vi "Auto.vi"   [LabVIEW 2017]
uses:
  <userlib>/836-Library/System/QCP_V2/QCPSupportCode/QCPData.ctl
  <userlib>/836-Library/System/QCP_V2/QCPSupportCode/QCP_GetDblArr.vi
  <userlib>/836-Library/System/QCP_V2/QCPSupportCode/QCP_GetDbl.vi
types:
  T1 = typedef "Semaphore RefNum" = refnum<k1>
  T2 = cluster{"Data Value Refnum":refnum<data-value>, "semaphore":T1}
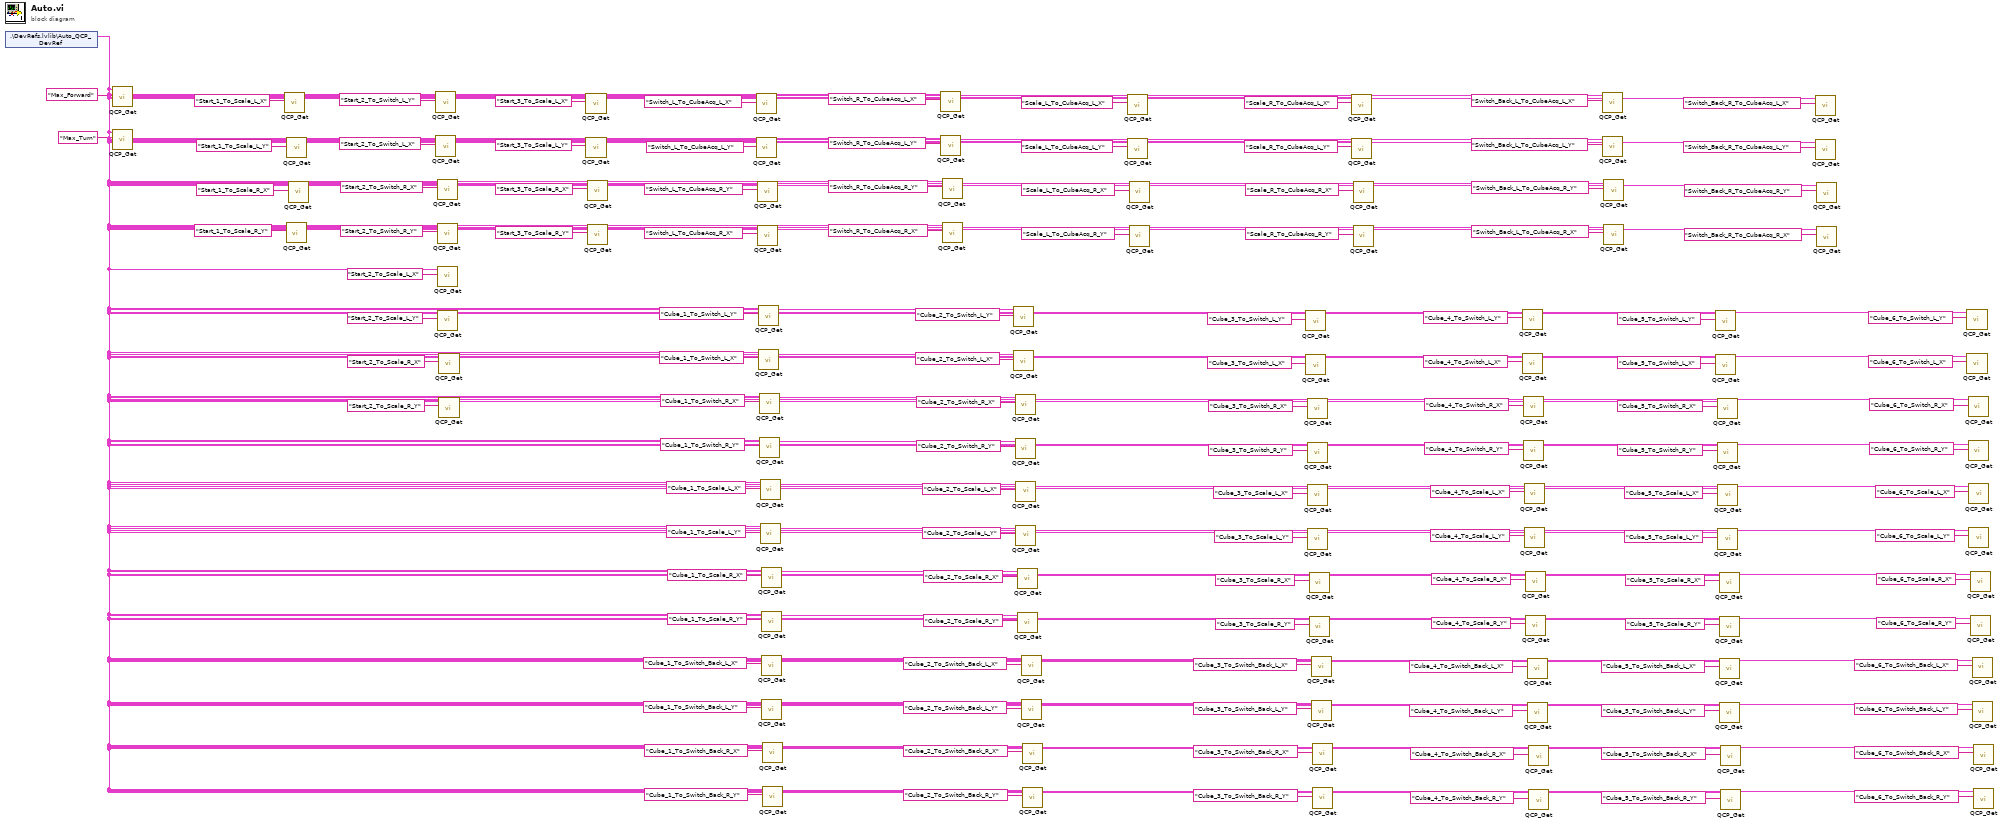
[diagram p0: block diagram]
diagram:
  n1 = shared-variable ".\\DevRefs.lvlib\\Auto_QCP_DevRef"() -> (w1:T2)  [unwired: 1 in, 1 out]
  n2 = call-poly <userlib>:"QCP_Get.vi"("Value Name"="Max_Forward", "QCP_DevRef_In"=w1) -> ()  [unwired: 7 in, 3 out]
  n3 = call-poly <userlib>:"QCP_Get.vi"("Value Name"="Max_Turn", "QCP_DevRef_In"=w1) -> ()  [unwired: 7 in, 3 out]
  n4 = call-poly <userlib>:"QCP_Get.vi"("Value Name"="Start_1_To_Scale_L_X", "QCP_DevRef_In"=w1) -> ()  [unwired: 7 in, 3 out]
  n5 = call-poly <userlib>:"QCP_Get.vi"("Value Name"="Start_1_To_Scale_R_Y", "QCP_DevRef_In"=w1) -> ()  [unwired: 7 in, 3 out]
  n6 = call-poly <userlib>:"QCP_Get.vi"("Value Name"="Start_1_To_Scale_L_Y", "QCP_DevRef_In"=w1) -> ()  [unwired: 7 in, 3 out]
  n7 = call-poly <userlib>:"QCP_Get.vi"("Value Name"="Start_1_To_Scale_R_X", "QCP_DevRef_In"=w1) -> ()  [unwired: 7 in, 3 out]
  n8 = call-poly <userlib>:"QCP_Get.vi"("Value Name"="Start_2_To_Switch_L_Y", "QCP_DevRef_In"=w1) -> ()  [unwired: 7 in, 3 out]
  n9 = call-poly <userlib>:"QCP_Get.vi"("Value Name"="Start_2_To_Switch_L_X", "QCP_DevRef_In"=w1) -> ()  [unwired: 7 in, 3 out]
  n10 = call-poly <userlib>:"QCP_Get.vi"("Value Name"="Start_2_To_Switch_R_X", "QCP_DevRef_In"=w1) -> ()  [unwired: 7 in, 3 out]
  n11 = call-poly <userlib>:"QCP_Get.vi"("Value Name"="Start_2_To_Switch_R_Y", "QCP_DevRef_In"=w1) -> ()  [unwired: 7 in, 3 out]
  n12 = call-poly <userlib>:"QCP_Get.vi"("Value Name"="Start_2_To_Scale_L_X", "QCP_DevRef_In"=w1) -> ()  [unwired: 7 in, 3 out]
  n13 = call-poly <userlib>:"QCP_Get.vi"("Value Name"="Start_2_To_Scale_L_Y", "QCP_DevRef_In"=w1) -> ()  [unwired: 7 in, 3 out]
  n14 = call-poly <userlib>:"QCP_Get.vi"("Value Name"="Start_2_To_Scale_R_X", "QCP_DevRef_In"=w1) -> ()  [unwired: 7 in, 3 out]
  n15 = call-poly <userlib>:"QCP_Get.vi"("Value Name"="Start_2_To_Scale_R_Y", "QCP_DevRef_In"=w1) -> ()  [unwired: 7 in, 3 out]
  n16 = call-poly <userlib>:"QCP_Get.vi"("Value Name"="Start_3_To_Scale_L_X", "QCP_DevRef_In"=w1) -> ()  [unwired: 7 in, 3 out]
  n17 = call-poly <userlib>:"QCP_Get.vi"("Value Name"="Start_3_To_Scale_L_Y", "QCP_DevRef_In"=w1) -> ()  [unwired: 7 in, 3 out]
  n18 = call-poly <userlib>:"QCP_Get.vi"("Value Name"="Start_3_To_Scale_R_X", "QCP_DevRef_In"=w1) -> ()  [unwired: 7 in, 3 out]
  n19 = call-poly <userlib>:"QCP_Get.vi"("Value Name"="Start_3_To_Scale_R_Y", "QCP_DevRef_In"=w1) -> ()  [unwired: 7 in, 3 out]
  n20 = call-poly <userlib>:"QCP_Get.vi"("Value Name"="Switch_L_To_CubeAcq_L_X", "QCP_DevRef_In"=w1) -> ()  [unwired: 7 in, 3 out]
  n21 = call-poly <userlib>:"QCP_Get.vi"("Value Name"="Switch_L_To_CubeAcq_L_Y", "QCP_DevRef_In"=w1) -> ()  [unwired: 7 in, 3 out]
  n22 = call-poly <userlib>:"QCP_Get.vi"("Value Name"="Switch_L_To_CubeAcq_R_Y", "QCP_DevRef_In"=w1) -> ()  [unwired: 7 in, 3 out]
  n23 = call-poly <userlib>:"QCP_Get.vi"("Value Name"="Switch_L_To_CubeAcq_R_X", "QCP_DevRef_In"=w1) -> ()  [unwired: 7 in, 3 out]
  n24 = call-poly <userlib>:"QCP_Get.vi"("Value Name"="Cube_1_To_Switch_L_Y", "QCP_DevRef_In"=w1) -> ()  [unwired: 7 in, 3 out]
  n25 = call-poly <userlib>:"QCP_Get.vi"("Value Name"="Cube_1_To_Switch_L_X", "QCP_DevRef_In"=w1) -> ()  [unwired: 7 in, 3 out]
  n26 = call-poly <userlib>:"QCP_Get.vi"("Value Name"="Cube_1_To_Switch_R_X", "QCP_DevRef_In"=w1) -> ()  [unwired: 7 in, 3 out]
  n27 = call-poly <userlib>:"QCP_Get.vi"("Value Name"="Cube_1_To_Switch_R_Y", "QCP_DevRef_In"=w1) -> ()  [unwired: 7 in, 3 out]
  n28 = call-poly <userlib>:"QCP_Get.vi"("Value Name"="Cube_1_To_Scale_L_X", "QCP_DevRef_In"=w1) -> ()  [unwired: 7 in, 3 out]
  n29 = call-poly <userlib>:"QCP_Get.vi"("Value Name"="Cube_1_To_Scale_L_Y", "QCP_DevRef_In"=w1) -> ()  [unwired: 7 in, 3 out]
  n30 = call-poly <userlib>:"QCP_Get.vi"("Value Name"="Cube_1_To_Scale_R_X", "QCP_DevRef_In"=w1) -> ()  [unwired: 7 in, 3 out]
  n31 = call-poly <userlib>:"QCP_Get.vi"("Value Name"="Cube_1_To_Scale_R_Y", "QCP_DevRef_In"=w1) -> ()  [unwired: 7 in, 3 out]
  n32 = call-poly <userlib>:"QCP_Get.vi"("Value Name"="Cube_1_To_Switch_Back_L_X", "QCP_DevRef_In"=w1) -> ()  [unwired: 7 in, 3 out]
  n33 = call-poly <userlib>:"QCP_Get.vi"("Value Name"="Cube_1_To_Switch_Back_L_Y", "QCP_DevRef_In"=w1) -> ()  [unwired: 7 in, 3 out]
  n34 = call-poly <userlib>:"QCP_Get.vi"("Value Name"="Cube_1_To_Switch_Back_R_X", "QCP_DevRef_In"=w1) -> ()  [unwired: 7 in, 3 out]
  n35 = call-poly <userlib>:"QCP_Get.vi"("Value Name"="Cube_1_To_Switch_Back_R_Y", "QCP_DevRef_In"=w1) -> ()  [unwired: 7 in, 3 out]
  n36 = call-poly <userlib>:"QCP_Get.vi"("Value Name"="Switch_R_To_CubeAcq_L_X", "QCP_DevRef_In"=w1) -> ()  [unwired: 7 in, 3 out]
  n37 = call-poly <userlib>:"QCP_Get.vi"("Value Name"="Switch_R_To_CubeAcq_L_Y", "QCP_DevRef_In"=w1) -> ()  [unwired: 7 in, 3 out]
  n38 = call-poly <userlib>:"QCP_Get.vi"("Value Name"="Switch_R_To_CubeAcq_R_Y", "QCP_DevRef_In"=w1) -> ()  [unwired: 7 in, 3 out]
  n39 = call-poly <userlib>:"QCP_Get.vi"("Value Name"="Switch_R_To_CubeAcq_R_X", "QCP_DevRef_In"=w1) -> ()  [unwired: 7 in, 3 out]
  n40 = call-poly <userlib>:"QCP_Get.vi"("Value Name"="Cube_2_To_Switch_L_Y", "QCP_DevRef_In"=w1) -> ()  [unwired: 7 in, 3 out]
  n41 = call-poly <userlib>:"QCP_Get.vi"("Value Name"="Cube_2_To_Switch_L_X", "QCP_DevRef_In"=w1) -> ()  [unwired: 7 in, 3 out]
  n42 = call-poly <userlib>:"QCP_Get.vi"("Value Name"="Cube_2_To_Switch_R_X", "QCP_DevRef_In"=w1) -> ()  [unwired: 7 in, 3 out]
  n43 = call-poly <userlib>:"QCP_Get.vi"("Value Name"="Cube_2_To_Switch_R_Y", "QCP_DevRef_In"=w1) -> ()  [unwired: 7 in, 3 out]
  n44 = call-poly <userlib>:"QCP_Get.vi"("Value Name"="Cube_2_To_Scale_L_X", "QCP_DevRef_In"=w1) -> ()  [unwired: 7 in, 3 out]
  n45 = call-poly <userlib>:"QCP_Get.vi"("Value Name"="Cube_2_To_Scale_L_Y", "QCP_DevRef_In"=w1) -> ()  [unwired: 7 in, 3 out]
  n46 = call-poly <userlib>:"QCP_Get.vi"("Value Name"="Cube_2_To_Scale_R_X", "QCP_DevRef_In"=w1) -> ()  [unwired: 7 in, 3 out]
  n47 = call-poly <userlib>:"QCP_Get.vi"("Value Name"="Cube_2_To_Scale_R_Y", "QCP_DevRef_In"=w1) -> ()  [unwired: 7 in, 3 out]
  n48 = call-poly <userlib>:"QCP_Get.vi"("Value Name"="Cube_2_To_Switch_Back_L_X", "QCP_DevRef_In"=w1) -> ()  [unwired: 7 in, 3 out]
  n49 = call-poly <userlib>:"QCP_Get.vi"("Value Name"="Cube_2_To_Switch_Back_L_Y", "QCP_DevRef_In"=w1) -> ()  [unwired: 7 in, 3 out]
  n50 = call-poly <userlib>:"QCP_Get.vi"("Value Name"="Cube_2_To_Switch_Back_R_X", "QCP_DevRef_In"=w1) -> ()  [unwired: 7 in, 3 out]
  n51 = call-poly <userlib>:"QCP_Get.vi"("Value Name"="Cube_2_To_Switch_Back_R_Y", "QCP_DevRef_In"=w1) -> ()  [unwired: 7 in, 3 out]
  n52 = call-poly <userlib>:"QCP_Get.vi"("Value Name"="Scale_L_To_CubeAcq_L_X", "QCP_DevRef_In"=w1) -> ()  [unwired: 7 in, 3 out]
  n53 = call-poly <userlib>:"QCP_Get.vi"("Value Name"="Scale_L_To_CubeAcq_L_Y", "QCP_DevRef_In"=w1) -> ()  [unwired: 7 in, 3 out]
  n54 = call-poly <userlib>:"QCP_Get.vi"("Value Name"="Scale_L_To_CubeAcq_R_X", "QCP_DevRef_In"=w1) -> ()  [unwired: 7 in, 3 out]
  n55 = call-poly <userlib>:"QCP_Get.vi"("Value Name"="Scale_L_To_CubeAcq_R_Y", "QCP_DevRef_In"=w1) -> ()  [unwired: 7 in, 3 out]
  n56 = call-poly <userlib>:"QCP_Get.vi"("Value Name"="Cube_3_To_Switch_L_Y", "QCP_DevRef_In"=w1) -> ()  [unwired: 7 in, 3 out]
  n57 = call-poly <userlib>:"QCP_Get.vi"("Value Name"="Cube_3_To_Switch_L_X", "QCP_DevRef_In"=w1) -> ()  [unwired: 7 in, 3 out]
  n58 = call-poly <userlib>:"QCP_Get.vi"("Value Name"="Cube_3_To_Switch_R_X", "QCP_DevRef_In"=w1) -> ()  [unwired: 7 in, 3 out]
  n59 = call-poly <userlib>:"QCP_Get.vi"("Value Name"="Cube_3_To_Switch_R_Y", "QCP_DevRef_In"=w1) -> ()  [unwired: 7 in, 3 out]
  n60 = call-poly <userlib>:"QCP_Get.vi"("Value Name"="Cube_3_To_Scale_L_X", "QCP_DevRef_In"=w1) -> ()  [unwired: 7 in, 3 out]
  n61 = call-poly <userlib>:"QCP_Get.vi"("Value Name"="Cube_3_To_Scale_L_Y", "QCP_DevRef_In"=w1) -> ()  [unwired: 7 in, 3 out]
  n62 = call-poly <userlib>:"QCP_Get.vi"("Value Name"="Cube_3_To_Scale_R_X", "QCP_DevRef_In"=w1) -> ()  [unwired: 7 in, 3 out]
  n63 = call-poly <userlib>:"QCP_Get.vi"("Value Name"="Cube_3_To_Scale_R_Y", "QCP_DevRef_In"=w1) -> ()  [unwired: 7 in, 3 out]
  n64 = call-poly <userlib>:"QCP_Get.vi"("Value Name"="Cube_3_To_Switch_Back_L_X", "QCP_DevRef_In"=w1) -> ()  [unwired: 7 in, 3 out]
  n65 = call-poly <userlib>:"QCP_Get.vi"("Value Name"="Cube_3_To_Switch_Back_L_Y", "QCP_DevRef_In"=w1) -> ()  [unwired: 7 in, 3 out]
  n66 = call-poly <userlib>:"QCP_Get.vi"("Value Name"="Cube_3_To_Switch_Back_R_X", "QCP_DevRef_In"=w1) -> ()  [unwired: 7 in, 3 out]
  n67 = call-poly <userlib>:"QCP_Get.vi"("Value Name"="Cube_3_To_Switch_Back_R_Y", "QCP_DevRef_In"=w1) -> ()  [unwired: 7 in, 3 out]
  n68 = call-poly <userlib>:"QCP_Get.vi"("Value Name"="Scale_R_To_CubeAcq_L_X", "QCP_DevRef_In"=w1) -> ()  [unwired: 7 in, 3 out]
  n69 = call-poly <userlib>:"QCP_Get.vi"("Value Name"="Scale_R_To_CubeAcq_L_Y", "QCP_DevRef_In"=w1) -> ()  [unwired: 7 in, 3 out]
  n70 = call-poly <userlib>:"QCP_Get.vi"("Value Name"="Scale_R_To_CubeAcq_R_X", "QCP_DevRef_In"=w1) -> ()  [unwired: 7 in, 3 out]
  n71 = call-poly <userlib>:"QCP_Get.vi"("Value Name"="Scale_R_To_CubeAcq_R_Y", "QCP_DevRef_In"=w1) -> ()  [unwired: 7 in, 3 out]
  n72 = call-poly <userlib>:"QCP_Get.vi"("Value Name"="Cube_4_To_Switch_L_Y", "QCP_DevRef_In"=w1) -> ()  [unwired: 7 in, 3 out]
  n73 = call-poly <userlib>:"QCP_Get.vi"("Value Name"="Cube_4_To_Switch_L_X", "QCP_DevRef_In"=w1) -> ()  [unwired: 7 in, 3 out]
  n74 = call-poly <userlib>:"QCP_Get.vi"("Value Name"="Cube_4_To_Switch_R_X", "QCP_DevRef_In"=w1) -> ()  [unwired: 7 in, 3 out]
  n75 = call-poly <userlib>:"QCP_Get.vi"("Value Name"="Cube_4_To_Switch_R_Y", "QCP_DevRef_In"=w1) -> ()  [unwired: 7 in, 3 out]
  n76 = call-poly <userlib>:"QCP_Get.vi"("Value Name"="Cube_4_To_Scale_L_X", "QCP_DevRef_In"=w1) -> ()  [unwired: 7 in, 3 out]
  n77 = call-poly <userlib>:"QCP_Get.vi"("Value Name"="Cube_4_To_Scale_L_Y", "QCP_DevRef_In"=w1) -> ()  [unwired: 7 in, 3 out]
  n78 = call-poly <userlib>:"QCP_Get.vi"("Value Name"="Cube_4_To_Scale_R_X", "QCP_DevRef_In"=w1) -> ()  [unwired: 7 in, 3 out]
  n79 = call-poly <userlib>:"QCP_Get.vi"("Value Name"="Cube_4_To_Scale_R_Y", "QCP_DevRef_In"=w1) -> ()  [unwired: 7 in, 3 out]
  n80 = call-poly <userlib>:"QCP_Get.vi"("Value Name"="Cube_4_To_Switch_Back_L_X", "QCP_DevRef_In"=w1) -> ()  [unwired: 7 in, 3 out]
  n81 = call-poly <userlib>:"QCP_Get.vi"("Value Name"="Cube_4_To_Switch_Back_L_Y", "QCP_DevRef_In"=w1) -> ()  [unwired: 7 in, 3 out]
  n82 = call-poly <userlib>:"QCP_Get.vi"("Value Name"="Cube_4_To_Switch_Back_R_X", "QCP_DevRef_In"=w1) -> ()  [unwired: 7 in, 3 out]
  n83 = call-poly <userlib>:"QCP_Get.vi"("Value Name"="Cube_4_To_Switch_Back_R_Y", "QCP_DevRef_In"=w1) -> ()  [unwired: 7 in, 3 out]
  n84 = call-poly <userlib>:"QCP_Get.vi"("Value Name"="Switch_Back_L_To_CubeAcq_L_X", "QCP_DevRef_In"=w1) -> ()  [unwired: 7 in, 3 out]
  n85 = call-poly <userlib>:"QCP_Get.vi"("Value Name"="Switch_Back_L_To_CubeAcq_L_Y", "QCP_DevRef_In"=w1) -> ()  [unwired: 7 in, 3 out]
  n86 = call-poly <userlib>:"QCP_Get.vi"("Value Name"="Switch_Back_L_To_CubeAcq_R_Y", "QCP_DevRef_In"=w1) -> ()  [unwired: 7 in, 3 out]
  n87 = call-poly <userlib>:"QCP_Get.vi"("Value Name"="Switch_Back_L_To_CubeAcq_R_X", "QCP_DevRef_In"=w1) -> ()  [unwired: 7 in, 3 out]
  n88 = call-poly <userlib>:"QCP_Get.vi"("Value Name"="Cube_5_To_Switch_L_Y", "QCP_DevRef_In"=w1) -> ()  [unwired: 7 in, 3 out]
  n89 = call-poly <userlib>:"QCP_Get.vi"("Value Name"="Cube_5_To_Switch_L_X", "QCP_DevRef_In"=w1) -> ()  [unwired: 7 in, 3 out]
  n90 = call-poly <userlib>:"QCP_Get.vi"("Value Name"="Cube_5_To_Switch_R_X", "QCP_DevRef_In"=w1) -> ()  [unwired: 7 in, 3 out]
  n91 = call-poly <userlib>:"QCP_Get.vi"("Value Name"="Cube_5_To_Switch_R_Y", "QCP_DevRef_In"=w1) -> ()  [unwired: 7 in, 3 out]
  n92 = call-poly <userlib>:"QCP_Get.vi"("Value Name"="Cube_5_To_Scale_L_X", "QCP_DevRef_In"=w1) -> ()  [unwired: 7 in, 3 out]
  n93 = call-poly <userlib>:"QCP_Get.vi"("Value Name"="Cube_5_To_Scale_L_Y", "QCP_DevRef_In"=w1) -> ()  [unwired: 7 in, 3 out]
  n94 = call-poly <userlib>:"QCP_Get.vi"("Value Name"="Cube_5_To_Scale_R_X", "QCP_DevRef_In"=w1) -> ()  [unwired: 7 in, 3 out]
  n95 = call-poly <userlib>:"QCP_Get.vi"("Value Name"="Cube_5_To_Scale_R_Y", "QCP_DevRef_In"=w1) -> ()  [unwired: 7 in, 3 out]
  n96 = call-poly <userlib>:"QCP_Get.vi"("Value Name"="Cube_5_To_Switch_Back_L_X", "QCP_DevRef_In"=w1) -> ()  [unwired: 7 in, 3 out]
  n97 = call-poly <userlib>:"QCP_Get.vi"("Value Name"="Cube_5_To_Switch_Back_L_Y", "QCP_DevRef_In"=w1) -> ()  [unwired: 7 in, 3 out]
  n98 = call-poly <userlib>:"QCP_Get.vi"("Value Name"="Cube_5_To_Switch_Back_R_X", "QCP_DevRef_In"=w1) -> ()  [unwired: 7 in, 3 out]
  n99 = call-poly <userlib>:"QCP_Get.vi"("Value Name"="Cube_5_To_Switch_Back_R_Y", "QCP_DevRef_In"=w1) -> ()  [unwired: 7 in, 3 out]
  n100 = call-poly <userlib>:"QCP_Get.vi"("Value Name"="Switch_Back_R_To_CubeAcq_L_X", "QCP_DevRef_In"=w1) -> ()  [unwired: 7 in, 3 out]
  n101 = call-poly <userlib>:"QCP_Get.vi"("Value Name"="Switch_Back_R_To_CubeAcq_L_Y", "QCP_DevRef_In"=w1) -> ()  [unwired: 7 in, 3 out]
  n102 = call-poly <userlib>:"QCP_Get.vi"("Value Name"="Switch_Back_R_To_CubeAcq_R_Y", "QCP_DevRef_In"=w1) -> ()  [unwired: 7 in, 3 out]
  n103 = call-poly <userlib>:"QCP_Get.vi"("Value Name"="Switch_Back_R_To_CubeAcq_R_X", "QCP_DevRef_In"=w1) -> ()  [unwired: 7 in, 3 out]
  n104 = call-poly <userlib>:"QCP_Get.vi"("Value Name"="Cube_6_To_Switch_L_Y", "QCP_DevRef_In"=w1) -> ()  [unwired: 7 in, 3 out]
  n105 = call-poly <userlib>:"QCP_Get.vi"("Value Name"="Cube_6_To_Switch_L_X", "QCP_DevRef_In"=w1) -> ()  [unwired: 7 in, 3 out]
  n106 = call-poly <userlib>:"QCP_Get.vi"("Value Name"="Cube_6_To_Switch_R_X", "QCP_DevRef_In"=w1) -> ()  [unwired: 7 in, 3 out]
  n107 = call-poly <userlib>:"QCP_Get.vi"("Value Name"="Cube_6_To_Switch_R_Y", "QCP_DevRef_In"=w1) -> ()  [unwired: 7 in, 3 out]
  n108 = call-poly <userlib>:"QCP_Get.vi"("Value Name"="Cube_6_To_Scale_L_X", "QCP_DevRef_In"=w1) -> ()  [unwired: 7 in, 3 out]
  n109 = call-poly <userlib>:"QCP_Get.vi"("Value Name"="Cube_6_To_Scale_L_Y", "QCP_DevRef_In"=w1) -> ()  [unwired: 7 in, 3 out]
  n110 = call-poly <userlib>:"QCP_Get.vi"("Value Name"="Cube_6_To_Scale_R_X", "QCP_DevRef_In"=w1) -> ()  [unwired: 7 in, 3 out]
  n111 = call-poly <userlib>:"QCP_Get.vi"("Value Name"="Cube_6_To_Scale_R_Y", "QCP_DevRef_In"=w1) -> ()  [unwired: 7 in, 3 out]
  n112 = call-poly <userlib>:"QCP_Get.vi"("Value Name"="Cube_6_To_Switch_Back_L_X", "QCP_DevRef_In"=w1) -> ()  [unwired: 7 in, 3 out]
  n113 = call-poly <userlib>:"QCP_Get.vi"("Value Name"="Cube_6_To_Switch_Back_L_Y", "QCP_DevRef_In"=w1) -> ()  [unwired: 7 in, 3 out]
  n114 = call-poly <userlib>:"QCP_Get.vi"("Value Name"="Cube_6_To_Switch_Back_R_X", "QCP_DevRef_In"=w1) -> ()  [unwired: 7 in, 3 out]
  n115 = call-poly <userlib>:"QCP_Get.vi"("Value Name"="Cube_6_To_Switch_Back_R_Y", "QCP_DevRef_In"=w1) -> ()  [unwired: 7 in, 3 out]
